vi "Write reinitializeIsTrue.vi"(10 "reinitializeIsTrue":bool, 11 "SystemController in":refnum<class "SystemController.lvclass">) -> (3 "SystemController out":refnum<class "SystemController.lvclass">)   [LabVIEW 2013, in "SystemController.lvclass"]
uses:
  SystemController.lvclass
  SystemController.lvclass/SystemController.ctl
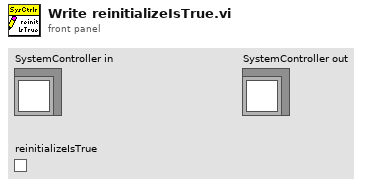
[diagram p1: front panel]
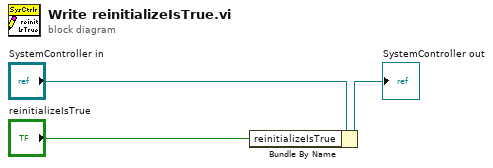
[diagram p0: block diagram]
diagram:
  n1 = Bundle By Name(cluster="SystemController in", "reinitializeIsTrue"="reinitializeIsTrue") -> (→"SystemController out":refnum<class "SystemController.lvclass">)
